vi "C_transfer_Q10_Z.vi"(3 "Qn":dbl[](array[numeric]) format="%#_13g", 4 "ek":dbl format="%#_13g") -> (1 "uk":dbl)   [LabVIEW 2015]
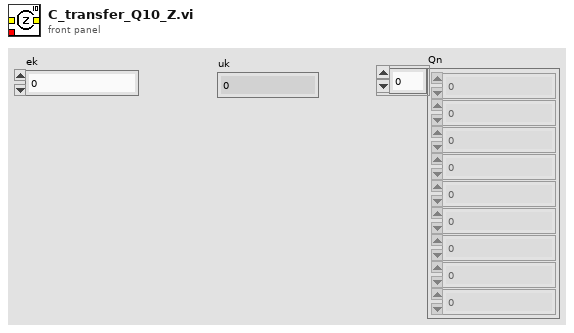
[diagram p1: front panel]
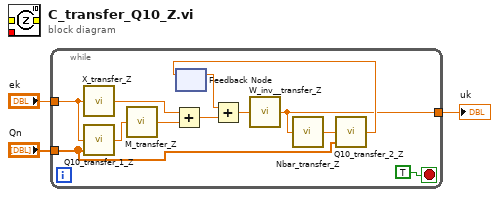
[diagram p0: block diagram]
diagram:
  n1 = while {
    tunnel: [w4] -> w3
    tunnel: "ek" -> [w11]
    tunnel: "Qn" -> [w6]
    stop <- TRUE stop-if-true
    n2 = call "X_transfer_Z.vi"("x"=w11) -> ("y"=w14:dbl)  [unwired: 4 in]
    n3 = call "Q10_transfer_1_Z.vi"("Qn"=w6, "x"=w11) -> ("y"=w13:dbl)  [unwired: 3 in]
    n4 = call "M_transfer_Z.vi"("x"=w13) -> ("y"=w12:dbl)  [unwired: 4 in]
    n5 = Add(x=w14, y=w12) -> (x+y=w8:dbl)
    n6 = feedback #1() -> (w7:dbl)  [unwired: 1 in]
    n7 = Add(x=w7, y=w8) -> (x+y=w10:dbl)
    n8 = call "W_inv__transfer_Z.vi"("x"=w10) -> ("y"=w4:dbl)  [unwired: 4 in]
    n9 = call "Nbar_transfer_Z.vi"("x"=w4) -> ("y"=w5:dbl)  [unwired: 4 in]
    n10 = call "Q10_transfer_2_Z .vi"("Qn"=w6, "x"=w5) -> ("y"=w9:dbl)  [unwired: 3 in]
    n11 = feedback-in #1(w9) -> ()
  }
  "uk" <- w3
